vi "Tidy and package_v00.vi"(0 "OPO A":T2={"Offset Error"=-0.08983050847457627, "Gain Error"=1, "Offset DC"=-0.003954802259887008, "Gain DC"=1, "P Gain"=20, "P Bit Shift"=-12, "I Bit Shift"=-12, "I2 Bit Shift"=-27, "I Gain"=20, "I2 Gain"=0, "Lock Threshold"=45, "Lock"=FALSE, "Hold"=FALSE, "Scan Frequency"=10, "Scan Bit Shift"=-4, "DC negative"=FALSE, "Gains -ve "=FALSE} {"Scan Frequency" scale=1.0..30.0; "I2 Gain" scale=0.0..10.0; "I Gain" scale=0.0..50.0; "P Gain" scale=0.0..50.0; "Offset DC" scale=-0.1..0.1 scale format="%#_5f"; "Offset Error" scale=-0.1..0.1 scale format="%#_5f"}, 5 "OPO B":T2={"Offset Error"=0.0, "Gain Error"=1, "Offset DC"=1.0, "Gain DC"=1, "P Gain"=20, "P Bit Shift"=-12, "I Bit Shift"=-12, "I2 Bit Shift"=-27, "I Gain"=20, "I2 Gain"=0, "Lock Threshold"=29, "Lock"=FALSE, "Hold"=TRUE, "Scan Frequency"=11, "Scan Bit Shift"=-4, "DC negative"=FALSE, "Gains -ve "=TRUE} {"Scan Frequency" scale=1.0..30.0; "I2 Gain" scale=0.0..10.0; "I Gain" scale=0.0..50.0; "P Gain" scale=0.0..50.0; "Offset DC" scale=-0.1..0.1 scale format="%#_5f"; "Offset Error" scale=-0.1..0.1 scale format="%#_5f"}, 7 "MCC":T2={"Offset Error"=0.0, "Gain Error"=1, "Offset DC"=0.0, "Gain DC"=1, "P Gain"=10, "P Bit Shift"=-12, "I Bit Shift"=-12, "I2 Bit Shift"=-27, "I Gain"=10, "I2 Gain"=0, "Lock Threshold"=16, "Lock"=FALSE, "Hold"=TRUE, "Scan Frequency"=10, "Scan Bit Shift"=-4, "DC negative"=FALSE, "Gains -ve "=TRUE} {"Scan Frequency" scale=1.0..30.0; "I2 Gain" scale=0.0..10.0; "I Gain" scale=0.0..50.0; "P Gain" scale=0.0..50.0; "Offset DC" scale=-0.1..0.1 scale format="%#_5f"; "Offset Error" scale=-0.1..0.1 scale format="%#_5f"}, 9 "Doubler":T2={"Offset Error"=-0.014124293785310736, "Gain Error"=1, "Offset DC"=0.011864406779661016, "Gain DC"=1, "P Gain"=11, "P Bit Shift"=-12, "I Bit Shift"=-12, "I2 Bit Shift"=-27, "I Gain"=13, "I2 Gain"=0, "Lock Threshold"=24, "Lock"=FALSE, "Hold"=TRUE, "Scan Frequency"=12, "Scan Bit Shift"=-4, "DC negative"=FALSE, "Gains -ve "=TRUE} {"Scan Frequency" scale=1.0..30.0; "I2 Gain" scale=0.0..10.0; "I Gain" scale=0.0..50.0; "P Gain" scale=0.0..50.0; "Offset DC" scale=-0.1..0.1 scale format="%#_5f"; "Offset Error" scale=-0.1..0.1 scale format="%#_5f"}, 11 "PII Controls (-1)":T19={"Safety First"={"lim reset"=FALSE, "no limit"=FALSE, "pos slew rate * dt"=40, "neg slew rate * dt"=-5, "Hold All"=FALSE, "Count(Ticks)"=0}, "Error scale"={"Bit Shift"={"Bit Shift 1"=2, "Bit Shift 2"=0, "Bit Shift 3"=0, "Bit Shift 4"=0, "Bit Shift 5"=2, "Bit Shift 6"=0, "Bit Shift 7"=0, "Bit Shift 8"=0}, "Pre-Offset"={"Pre-Offset 1"=0, "Pre-Offset 2"=300, "Pre-Offset 3"=0, "Pre-Offset 4"=0, "Pre-Offset 5"=0, "Pre-Offset 6"=0, "Pre-Offset 7"=0, "Pre-Offset 8"=0}, "Post-Offset "={"Offset 1"=0, "Offset 2"=300, "Offset 3"=0, "Offset 4"=0, "Offset 5"=0, "Offset 6"=0, "Offset 7"=0, "Offset 8"=0}, "Gains"={"Gain 1"=5, "Gain 2"=5, "Gain 3"=0, "Gain 4"=0, "Gain 5"=0, "Gain 6"=0, "Gain 7"=0, "Gain 8"=0}, "Polarity DC"={"False 1"=FALSE, "False 2"=FALSE, "False 3"=FALSE, "False 4"=FALSE, "DC x -1"=FALSE, "DC x -1 2"=FALSE, "DC x -1 3"=FALSE, "DC x -1 4"=FALSE}}, "Lock Select"=enum."OPO A", "Controls"={"OPO A"={"Pre Offset"=0.0, "Offset"=0.0, "Gain"=0, "Bit Shift"=0, "Pre Offset 2"=0.0, "Offset 2"=0.0, "Gain 2"=0, "Bit Shift 2"=0, "P Gain"=0, "P Bit Shift"=0, "I Bit Shift"=0, "I2 Bit Shift"=0, "I Gain"=0, "I2 Gain"=0, "Lock Threshold"=0, "Lock"=FALSE, "Hold"=FALSE, "Scan Offset (mV)"=0.0, "Scan Amplitude (mV)"=0.0, "Scan Frequency"=0, "Scan Bit Shift"=0, "DC x -1"=FALSE, "Gains x -1"=FALSE, "I Max value"=0, "I2 Max value"=0}, "OPO B"={"Pre Offset"=0.0, "Offset"=0.0, "Gain"=0, "Bit Shift"=0, "Pre Offset 2"=0.0, "Offset 2"=0.0, "Gain 2"=0, "Bit Shift 2"=0, "P Gain"=0, "P Bit Shift"=0, "I Bit Shift"=0, "I2 Bit Shift"=0, "I Gain"=0, "I2 Gain"=0, "Lock Threshold"=0, "Lock"=FALSE, "Hold"=FALSE, "Scan Offset (mV)"=0.0, "Scan Amplitude (mV)"=0.0, "Scan Frequency"=0, "Scan Bit Shift"=0, "DC x -1"=FALSE, "Gains x -1"=FALSE, "I Max value"=0, "I2 Max value"=0}, "MCC"={"Pre Offset"=0.0, "Offset"=0.0, "Gain"=0, "Bit Shift"=0, "Pre Offset 2"=0.0, "Offset 2"=0.0, "Gain 2"=0, "Bit Shift 2"=0, "P Gain"=0, "P Bit Shift"=0, "I Bit Shift"=0, "I2 Bit Shift"=0, "I Gain"=0, "I2 Gain"=0, "Lock Threshold"=0, "Lock"=FALSE, "Hold"=FALSE, "Scan Offset (mV)"=0.0, "Scan Amplitude (mV)"=0.0, "Scan Frequency"=0, "Scan Bit Shift"=0, "DC x -1"=FALSE, "Gains x -1"=FALSE, "I Max value"=0, "I2 Max value"=0}, "Doubler"={"Pre Offset"=0.0, "Offset"=0.0, "Gain"=0, "Bit Shift"=0, "Pre Offset 2"=0.0, "Offset 2"=0.0, "Gain 2"=0, "Bit Shift 2"=0, "P Gain"=0, "P Bit Shift"=0, "I Bit Shift"=0, "I2 Bit Shift"=0, "I Gain"=0, "I2 Gain"=0, "Lock Threshold"=0, "Lock"=FALSE, "Hold"=FALSE, "Scan Offset (mV)"=0.0, "Scan Amplitude (mV)"=0.0, "Scan Frequency"=0, "Scan Bit Shift"=0, "DC x -1"=FALSE, "Gains x -1"=FALSE, "I Max value"=0, "I2 Max value"=0}}, "Scope IPs"={"Trigger Direction"=enum."either", "Trigger Delay (ms)"=0.0, "Aquisition Rate (kHz)"=1.0, "Trigger Offset (V)"=-1.0, "Trigger Channel"=0, "Channel Selector"={"Channel 1"=0, "Channel 2"=0, "Channel 3"=0, "Channel 4"=0}, "Scale Offset"={"Scaling"={"Scan Scale"=0, "Scan Scale 2"=0, "Scan Scale 3"=0, "Scan Scale 4"=0}, "Offset"={"Scan Offset"=0, "Scan Offset 2"=0, "Scan Offset 3"=0, "Scan Offset 4"=0}}}, "PII A"={"Lock"=FALSE, "Hold"=FALSE, "P Gain"=0, "P BS"=0, "I Gain"=0, "I BS"=0, "I2 G"=0, "I2 BS"=0, "Scan Amp"=0, "Scan Off"=0, "Scan FS"=0, "SFS BS"=0, "I Max value"=0, "I2 Max value"=0}, "PII B"={"Lock"=FALSE, "Hold"=FALSE, "P Gain"=0, "P BS"=0, "I Gain"=0, "I BS"=0, "I2 G"=0, "I2 BS"=0, "Scan Amp"=0, "Scan Off"=0, "Scan FS"=0, "SFS BS"=0, "I Max value"=0, "I2 Max value"=0}, "PII MCC"={"Lock"=FALSE, "Hold"=FALSE, "P Gain"=0, "P BS"=0, "I Gain"=0, "I BS"=0, "I2 G"=0, "I2 BS"=0, "Scan Amp"=0, "Scan Off"=0, "Scan FS"=0, "SFS BS"=0, "I Max value"=0, "I2 Max value"=0}, "PII Doubler"={"Lock"=FALSE, "Hold"=FALSE, "P Gain"=0, "P BS"=0, "I Gain"=0, "I BS"=0, "I2 G"=0, "I2 BS"=0, "Scan Amp"=0, "Scan Off"=0, "Scan FS"=0, "SFS BS"=0, "I Max value"=0, "I2 Max value"=0}, "Peak Depth (%)"={"Peak Depth (%) 1"=0, "Peak Depth (%) 2"=0, "Peak Depth (%) 3"=0, "Peak Depth (%) 4"=0}} {"Controls"."OPO A"."Scan Bit Shift" min=-8 max=0; "Controls"."OPO A"."Scan Frequency" scale=1.0..30.0; "Controls"."OPO A"."Scan Amplitude (mV)" scale=100.0..3000.0 scale format="%#_5f"; "Controls"."OPO A"."Scan Offset (mV)" scale=100.0..3000.0 scale format="%#_5f"; "Controls"."OPO A"."I2 Gain" scale=0.0..50.0; "Controls"."OPO A"."I Gain" scale=0.0..50.0; "Controls"."OPO A"."P Gain" scale=0.0..50.0; "Controls"."OPO A"."Offset 2" scale=-0.1..0.1 scale format="%#_5f"; "Controls"."OPO A"."Pre Offset 2" scale=-0.1..0.1 scale format="%#_5f"; "Controls"."OPO A"."Offset" scale=-0.1..0.1 scale format="%#_5f"; "Controls"."OPO A"."Pre Offset" scale=-0.1..0.1 scale format="%#_5f"; "Controls"."OPO B"."Scan Bit Shift" min=-8 max=0; "Controls"."OPO B"."Scan Frequency" scale=1.0..30.0; "Controls"."OPO B"."Scan Amplitude (mV)" scale=100.0..3000.0 scale format="%#_5f"; "Controls"."OPO B"."Scan Offset (mV)" scale=100.0..3000.0 scale format="%#_5f"; "Controls"."OPO B"."I2 Gain" scale=0.0..50.0; "Controls"."OPO B"."I Gain" scale=0.0..50.0; "Controls"."OPO B"."P Gain" scale=0.0..50.0; "Controls"."OPO B"."Offset 2" scale=-0.1..0.1 scale format="%#_5f"; "Controls"."OPO B"."Pre Offset 2" scale=-0.1..0.1 scale format="%#_5f"; "Controls"."OPO B"."Offset" scale=-0.1..0.1 scale format="%#_5f"; "Controls"."OPO B"."Pre Offset" scale=-0.1..0.1 scale format="%#_5f"; "Controls"."MCC"."Scan Bit Shift" min=-8 max=0; "Controls"."MCC"."Scan Frequency" scale=1.0..30.0; "Controls"."MCC"."Scan Amplitude (mV)" scale=100.0..3000.0 scale format="%#_5f"; "Controls"."MCC"."Scan Offset (mV)" scale=100.0..3000.0 scale format="%#_5f"; "Controls"."MCC"."I2 Gain" scale=0.0..50.0; "Controls"."MCC"."I Gain" scale=0.0..50.0; "Controls"."MCC"."P Gain" scale=0.0..50.0; "Controls"."MCC"."Offset 2" scale=-0.1..0.1 scale format="%#_5f"; "Controls"."MCC"."Pre Offset 2" scale=-0.1..0.1 scale format="%#_5f"; "Controls"."MCC"."Offset" scale=-0.1..0.1 scale format="%#_5f"; "Controls"."MCC"."Pre Offset" scale=-0.1..0.1 scale format="%#_5f"; "Controls"."Doubler"."Scan Bit Shift" min=-8 max=0; "Controls"."Doubler"."Scan Frequency" scale=1.0..30.0; "Controls"."Doubler"."Scan Amplitude (mV)" scale=100.0..3000.0 scale format="%#_5f"; "Controls"."Doubler"."Scan Offset (mV)" scale=100.0..3000.0 scale format="%#_5f"; "Controls"."Doubler"."I2 Gain" scale=0.0..50.0; "Controls"."Doubler"."I Gain" scale=0.0..50.0; "Controls"."Doubler"."P Gain" scale=0.0..50.0; "Controls"."Doubler"."Offset 2" scale=-0.1..0.1 scale format="%#_5f"; "Controls"."Doubler"."Pre Offset 2" scale=-0.1..0.1 scale format="%#_5f"; "Controls"."Doubler"."Offset" scale=-0.1..0.1 scale format="%#_5f"; "Controls"."Doubler"."Pre Offset" scale=-0.1..0.1 scale format="%#_5f"}, 12 "Cavity Extras":T16={"Pre-Offset"={"OPO A"=0.0, "OPO B"=0.0, "MCC"=0.0, "Doubler"=0.0}, "Pre-Offset DC"={"OPO A"=0.0, "OPO B"=0.0, "MCC"=0.0, "Doubler"=0.0}, "I Max value"=20000, "I2 Max value"=20000, "Scan Offset"={"OPO A"=0.0, "OPO B"=0.0, "MCC"=0.0, "Doubler"=0.0}, "Scan Ampl."={"OPO A"=1000.0, "OPO B"=1000.0, "MCC"=1000.0, "Doubler"=1000.0}, "Scan-PII thresh"={"OPO A"=0, "OPO B"=0, "MCC"=0, "Doubler"=0}, "Re-Scan thresh"={"OPO A"=0, "OPO B"=0, "MCC"=0, "Doubler"=0}}, 13 "Scope+Safety":T15={"Safety First"={"lim reset"=FALSE, "no limit"=FALSE, "pos slew rate * dt"=100, "neg slew rate * dt"=-100, "Count(Ticks)"=0}, "Scope IPs"={"Trigger Direction"=enum."minus-plus", "Trigger Delay (ms)"=0.0, "Aquisition Rate (kHz)"=4000.0, "Trigger Offset (V)"=0.0, "Scale Offset"={"Scaling"={"Error signal"=1, "Output"=1, "DC Monitor"=1, "Threshold"=1}, "Offset"={"Error Signal"=0, "Output"=0, "DC Monitor"=0, "Threshold"=0}}}}, 14 "Hold All":T12) -> (3 "PII Controls cluster":T19={"Safety First"={"lim reset"=FALSE, "no limit"=FALSE, "pos slew rate * dt"=40, "neg slew rate * dt"=-5, "Hold All"=FALSE, "Count(Ticks)"=0}, "Error scale"={"Bit Shift"={"Bit Shift 1"=2, "Bit Shift 2"=0, "Bit Shift 3"=0, "Bit Shift 4"=0, "Bit Shift 5"=2, "Bit Shift 6"=0, "Bit Shift 7"=0, "Bit Shift 8"=0}, "Pre-Offset"={"Pre-Offset 1"=0, "Pre-Offset 2"=300, "Pre-Offset 3"=0, "Pre-Offset 4"=0, "Pre-Offset 5"=0, "Pre-Offset 6"=0, "Pre-Offset 7"=0, "Pre-Offset 8"=0}, "Post-Offset "={"Offset 1"=0, "Offset 2"=300, "Offset 3"=0, "Offset 4"=0, "Offset 5"=0, "Offset 6"=0, "Offset 7"=0, "Offset 8"=0}, "Gains"={"Gain 1"=5, "Gain 2"=5, "Gain 3"=0, "Gain 4"=0, "Gain 5"=0, "Gain 6"=0, "Gain 7"=0, "Gain 8"=0}, "Polarity DC"={"False 1"=FALSE, "False 2"=FALSE, "False 3"=FALSE, "False 4"=FALSE, "DC x -1"=FALSE, "DC x -1 2"=FALSE, "DC x -1 3"=FALSE, "DC x -1 4"=FALSE}}, "Lock Select"=enum."OPO A", "Controls"={"OPO A"={"Pre Offset"=0.0, "Offset"=0.0, "Gain"=0, "Bit Shift"=0, "Pre Offset 2"=0.0, "Offset 2"=0.0, "Gain 2"=0, "Bit Shift 2"=0, "P Gain"=0, "P Bit Shift"=0, "I Bit Shift"=0, "I2 Bit Shift"=0, "I Gain"=0, "I2 Gain"=0, "Lock Threshold"=0, "Lock"=FALSE, "Hold"=FALSE, "Scan Offset (mV)"=0.0, "Scan Amplitude (mV)"=0.0, "Scan Frequency"=0, "Scan Bit Shift"=0, "DC x -1"=FALSE, "Gains x -1"=FALSE, "I Max value"=0, "I2 Max value"=0}, "OPO B"={"Pre Offset"=0.0, "Offset"=0.0, "Gain"=0, "Bit Shift"=0, "Pre Offset 2"=0.0, "Offset 2"=0.0, "Gain 2"=0, "Bit Shift 2"=0, "P Gain"=0, "P Bit Shift"=0, "I Bit Shift"=0, "I2 Bit Shift"=0, "I Gain"=0, "I2 Gain"=0, "Lock Threshold"=0, "Lock"=FALSE, "Hold"=FALSE, "Scan Offset (mV)"=0.0, "Scan Amplitude (mV)"=0.0, "Scan Frequency"=0, "Scan Bit Shift"=0, "DC x -1"=FALSE, "Gains x -1"=FALSE, "I Max value"=0, "I2 Max value"=0}, "MCC"={"Pre Offset"=0.0, "Offset"=0.0, "Gain"=0, "Bit Shift"=0, "Pre Offset 2"=0.0, "Offset 2"=0.0, "Gain 2"=0, "Bit Shift 2"=0, "P Gain"=0, "P Bit Shift"=0, "I Bit Shift"=0, "I2 Bit Shift"=0, "I Gain"=0, "I2 Gain"=0, "Lock Threshold"=0, "Lock"=FALSE, "Hold"=FALSE, "Scan Offset (mV)"=0.0, "Scan Amplitude (mV)"=0.0, "Scan Frequency"=0, "Scan Bit Shift"=0, "DC x -1"=FALSE, "Gains x -1"=FALSE, "I Max value"=0, "I2 Max value"=0}, "Doubler"={"Pre Offset"=0.0, "Offset"=0.0, "Gain"=0, "Bit Shift"=0, "Pre Offset 2"=0.0, "Offset 2"=0.0, "Gain 2"=0, "Bit Shift 2"=0, "P Gain"=0, "P Bit Shift"=0, "I Bit Shift"=0, "I2 Bit Shift"=0, "I Gain"=0, "I2 Gain"=0, "Lock Threshold"=0, "Lock"=FALSE, "Hold"=FALSE, "Scan Offset (mV)"=0.0, "Scan Amplitude (mV)"=0.0, "Scan Frequency"=0, "Scan Bit Shift"=0, "DC x -1"=FALSE, "Gains x -1"=FALSE, "I Max value"=0, "I2 Max value"=0}}, "Scope IPs"={"Trigger Direction"=enum."either", "Trigger Delay (ms)"=0.0, "Aquisition Rate (kHz)"=1.0, "Trigger Offset (V)"=-1.0, "Trigger Channel"=0, "Channel Selector"={"Channel 1"=0, "Channel 2"=0, "Channel 3"=0, "Channel 4"=0}, "Scale Offset"={"Scaling"={"Scan Scale"=0, "Scan Scale 2"=0, "Scan Scale 3"=0, "Scan Scale 4"=0}, "Offset"={"Scan Offset"=0, "Scan Offset 2"=0, "Scan Offset 3"=0, "Scan Offset 4"=0}}}, "PII A"={"Lock"=FALSE, "Hold"=FALSE, "P Gain"=0, "P BS"=0, "I Gain"=0, "I BS"=0, "I2 G"=0, "I2 BS"=0, "Scan Amp"=0, "Scan Off"=0, "Scan FS"=0, "SFS BS"=0, "I Max value"=0, "I2 Max value"=0}, "PII B"={"Lock"=FALSE, "Hold"=FALSE, "P Gain"=0, "P BS"=0, "I Gain"=0, "I BS"=0, "I2 G"=0, "I2 BS"=0, "Scan Amp"=0, "Scan Off"=0, "Scan FS"=0, "SFS BS"=0, "I Max value"=0, "I2 Max value"=0}, "PII MCC"={"Lock"=FALSE, "Hold"=FALSE, "P Gain"=0, "P BS"=0, "I Gain"=0, "I BS"=0, "I2 G"=0, "I2 BS"=0, "Scan Amp"=0, "Scan Off"=0, "Scan FS"=0, "SFS BS"=0, "I Max value"=0, "I2 Max value"=0}, "PII Doubler"={"Lock"=FALSE, "Hold"=FALSE, "P Gain"=0, "P BS"=0, "I Gain"=0, "I BS"=0, "I2 G"=0, "I2 BS"=0, "Scan Amp"=0, "Scan Off"=0, "Scan FS"=0, "SFS BS"=0, "I Max value"=0, "I2 Max value"=0}, "Peak Depth (%)"={"Peak Depth (%) 1"=0, "Peak Depth (%) 2"=0, "Peak Depth (%) 3"=0, "Peak Depth (%) 4"=0}} {"Controls"."OPO A"."Scan Bit Shift" min=-8 max=0; "Controls"."OPO A"."Scan Frequency" scale=1.0..30.0; "Controls"."OPO A"."Scan Amplitude (mV)" scale=100.0..3000.0 scale format="%#_5f"; "Controls"."OPO A"."Scan Offset (mV)" scale=100.0..3000.0 scale format="%#_5f"; "Controls"."OPO A"."I2 Gain" scale=0.0..50.0; "Controls"."OPO A"."I Gain" scale=0.0..50.0; "Controls"."OPO A"."P Gain" scale=0.0..50.0; "Controls"."OPO A"."Offset 2" scale=-0.1..0.1 scale format="%#_5f"; "Controls"."OPO A"."Pre Offset 2" scale=-0.1..0.1 scale format="%#_5f"; "Controls"."OPO A"."Offset" scale=-0.1..0.1 scale format="%#_5f"; "Controls"."OPO A"."Pre Offset" scale=-0.1..0.1 scale format="%#_5f"; "Controls"."OPO B"."Scan Bit Shift" min=-8 max=0; "Controls"."OPO B"."Scan Frequency" scale=1.0..30.0; "Controls"."OPO B"."Scan Amplitude (mV)" scale=100.0..3000.0 scale format="%#_5f"; "Controls"."OPO B"."Scan Offset (mV)" scale=100.0..3000.0 scale format="%#_5f"; "Controls"."OPO B"."I2 Gain" scale=0.0..50.0; "Controls"."OPO B"."I Gain" scale=0.0..50.0; "Controls"."OPO B"."P Gain" scale=0.0..50.0; "Controls"."OPO B"."Offset 2" scale=-0.1..0.1 scale format="%#_5f"; "Controls"."OPO B"."Pre Offset 2" scale=-0.1..0.1 scale format="%#_5f"; "Controls"."OPO B"."Offset" scale=-0.1..0.1 scale format="%#_5f"; "Controls"."OPO B"."Pre Offset" scale=-0.1..0.1 scale format="%#_5f"; "Controls"."MCC"."Scan Bit Shift" min=-8 max=0; "Controls"."MCC"."Scan Frequency" scale=1.0..30.0; "Controls"."MCC"."Scan Amplitude (mV)" scale=100.0..3000.0 scale format="%#_5f"; "Controls"."MCC"."Scan Offset (mV)" scale=100.0..3000.0 scale format="%#_5f"; "Controls"."MCC"."I2 Gain" scale=0.0..50.0; "Controls"."MCC"."I Gain" scale=0.0..50.0; "Controls"."MCC"."P Gain" scale=0.0..50.0; "Controls"."MCC"."Offset 2" scale=-0.1..0.1 scale format="%#_5f"; "Controls"."MCC"."Pre Offset 2" scale=-0.1..0.1 scale format="%#_5f"; "Controls"."MCC"."Offset" scale=-0.1..0.1 scale format="%#_5f"; "Controls"."MCC"."Pre Offset" scale=-0.1..0.1 scale format="%#_5f"; "Controls"."Doubler"."Scan Bit Shift" min=-8 max=0; "Controls"."Doubler"."Scan Frequency" scale=1.0..30.0; "Controls"."Doubler"."Scan Amplitude (mV)" scale=100.0..3000.0 scale format="%#_5f"; "Controls"."Doubler"."Scan Offset (mV)" scale=100.0..3000.0 scale format="%#_5f"; "Controls"."Doubler"."I2 Gain" scale=0.0..50.0; "Controls"."Doubler"."I Gain" scale=0.0..50.0; "Controls"."Doubler"."P Gain" scale=0.0..50.0; "Controls"."Doubler"."Offset 2" scale=-0.1..0.1 scale format="%#_5f"; "Controls"."Doubler"."Pre Offset 2" scale=-0.1..0.1 scale format="%#_5f"; "Controls"."Doubler"."Offset" scale=-0.1..0.1 scale format="%#_5f"; "Controls"."Doubler"."Pre Offset" scale=-0.1..0.1 scale format="%#_5f"}, 4 "Scope IPs":T13, 15 "Control to FPGA":T18)   [LabVIEW 2010]
doc: "The data structures from the User Interface need are rebundled here to match that of the FPGA_Cavity VI."
uses:
  Strict Type Defs/Top Level Control.ctl
  Strict Type Defs/Safety First.ctl
  Strict Type Defs/Error_Scale.ctl
  Strict Type Defs/Control GUI v00.ctl
  Strict Type Defs/Slider and display.ctl
  Strict Type Defs/I16 white control.ctl
  Strict Type Defs/PII Gains.ctl
  Strict Type Defs/Thresh slider.ctl
  Strict Type Defs/Lock or Hold.ctl
  Strict Type Defs/Scan Amp slider.ctl
  Strict Type Defs/Scan Frequency.ctl
  Strict Type Defs/DC polarity.ctl
  Strict Type Defs/Gains negative.ctl
  Strict Type Defs/I max value.ctl
  Strict Type Defs/Top Level PII.ctl
  Strict Type Defs/Control GUI v01.ctl
  Strict Type Defs/I2 gain slider.ctl
  Strict Type Defs/Scan Freq Slider.ctl
  Strict Type Defs/Gains negative vertical.ctl
  Strict Type Defs/Cavity Extras.ctl
  Strict Type Defs/Pre-Offset.ctl
  Strict Type Defs/Scope and Safety.ctl
  Strict Type Defs/Hold All.ctl
  Strict Type Defs/Lock Select 4.ctl
panel:
  in  "Lock 4":T1
  in  "Safety First":T14
  in  "Control":T18
  # "PII Gains"
  # "Lock"
  # "Error Signal"
  # "Monitor"
  # "Scan"
  # "DC positive"
  # "PII Gains"
  # "Lock"
  # "Error Signal"
  # "Monitor"
  # "Scan"
  # "DC positive"
  # "PII Gains"
  # "Lock"
  # "Error Signal"
  # "Monitor"
  # "Scan"
  # "DC positive"
  # "PII Gains"
  # "Lock"
  # "Error Signal"
  # "Monitor"
  # "Scan"
  # "DC positive"
  # "Error Signal"
  # "Cavity Monitors"
  # "PII Gains"
  # "Lock"
  # "Scan"
  # "Error Signal"
  # "Cavity Monitors"
  # "PII Gains"
  # "Lock"
  # "Scan"
  # "Error Signal"
  # "Cavity Monitors"
  # "PII Gains"
  # "Lock"
  # "Scan"
  # "Error Signal"
  # "Cavity Monitors"
  # "PII Gains"
  # "Lock"
  # "Scan"
  # "Error Signal"
  # "Cavity Monitors"
  # "PII Gains"
  # "Lock"
  # "Scan"
  # "Error Signal"
  # "Cavity Monitors"
  # "PII Gains"
  # "Lock"
  # "Scan"
  # "Error Signal"
  # "Cavity Monitors"
  # "PII Gains"
  # "Lock"
  # "Scan"
  # "Error Signal"
  # "Cavity Monitors"
  # "PII Gains"
  # "Lock"
  # "Scan"
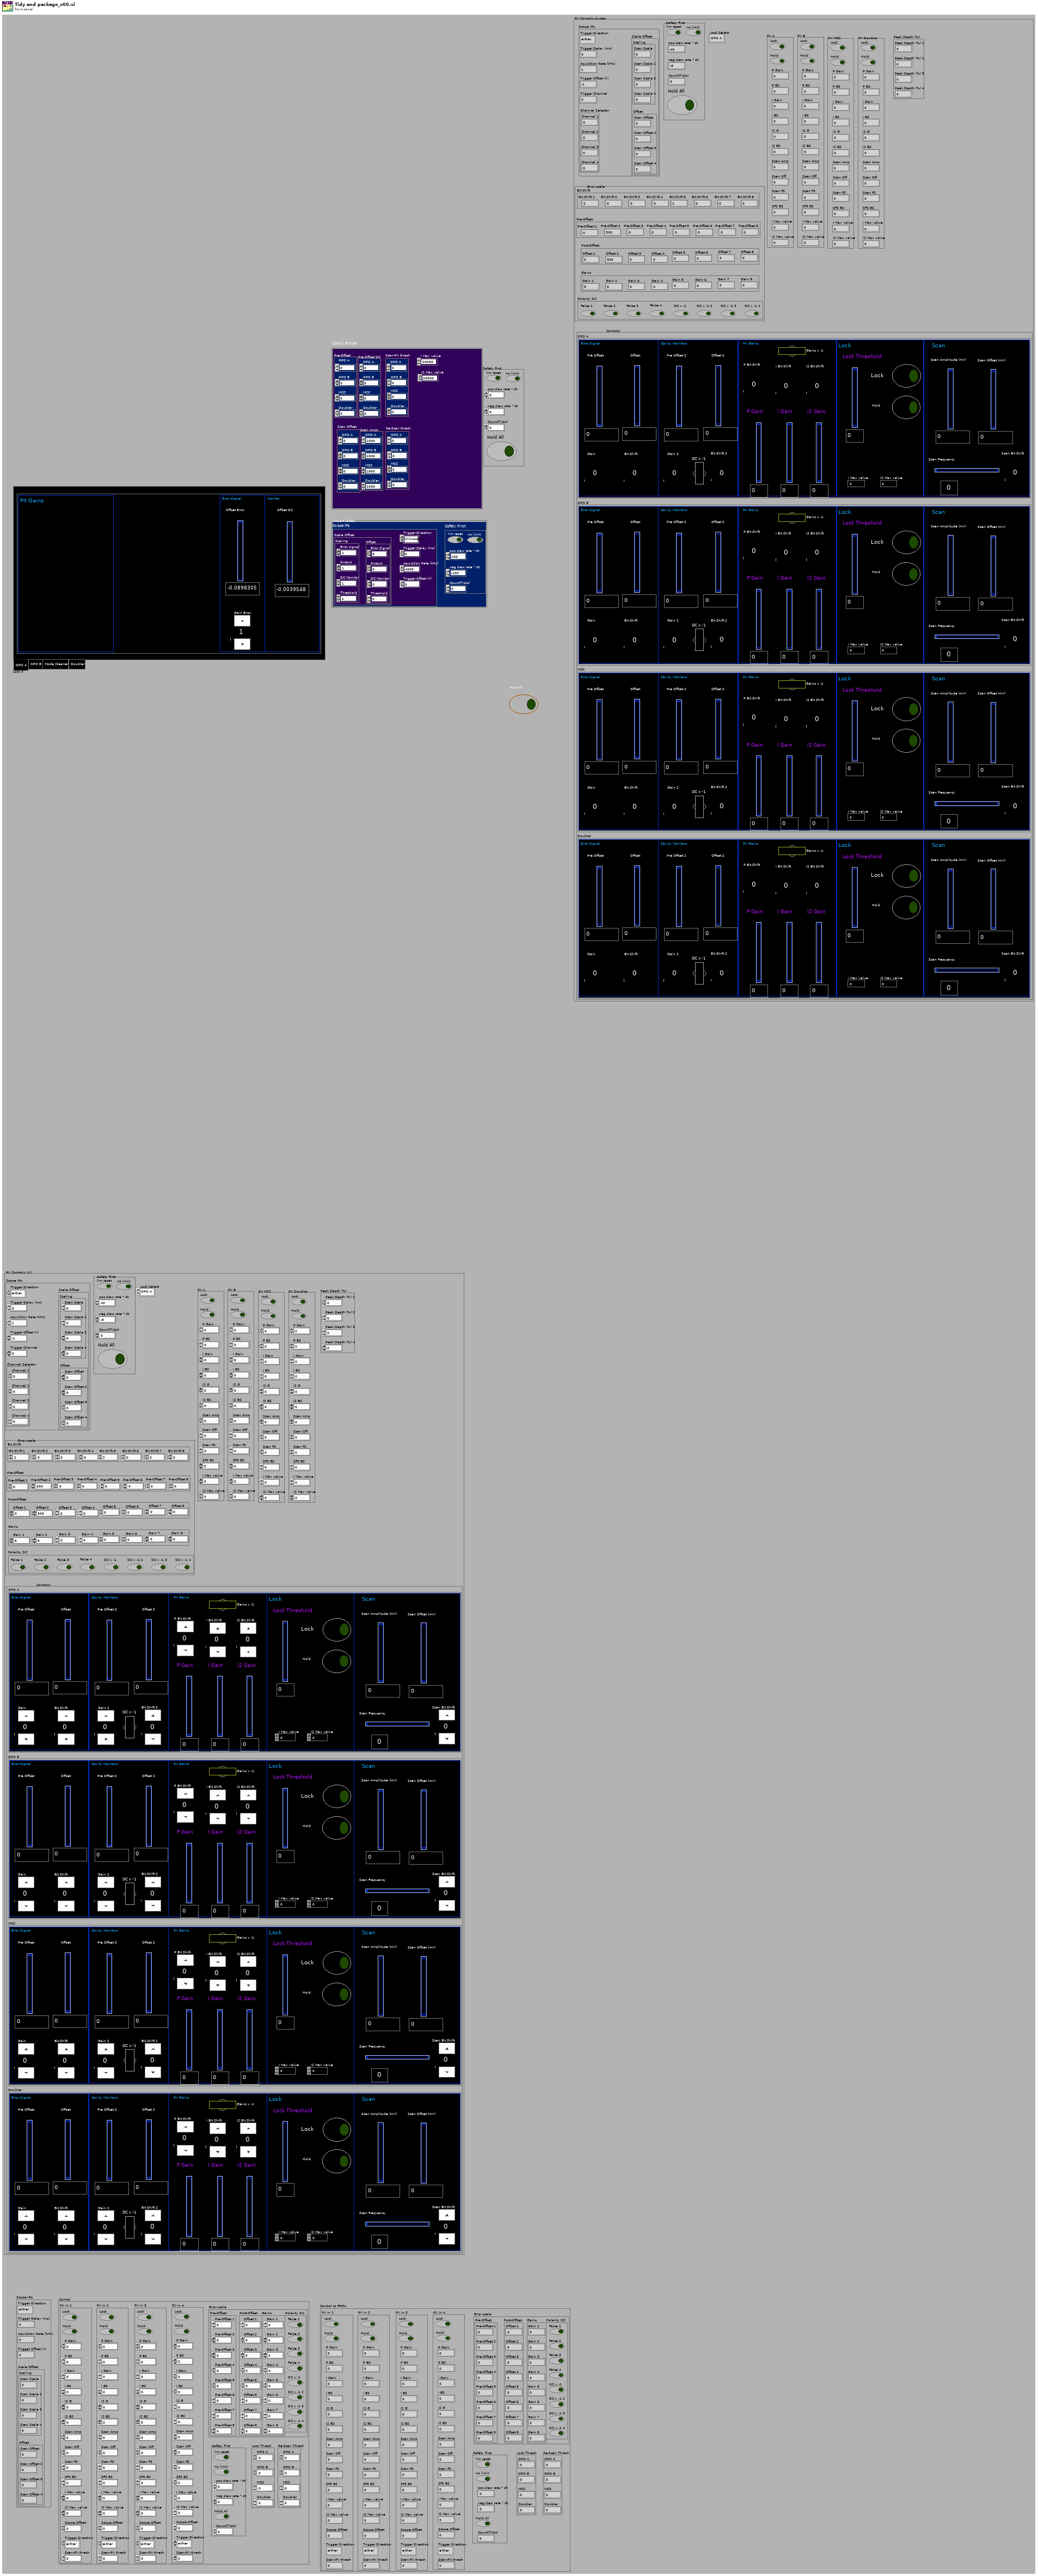
[diagram p1: front panel]
types:
  T1 = typedef "Lock Select 4.ctl" = enum32{"OPO A", "OPO B", "Mode Cleaner", "Doubler"}
  T2 = typedef "Control GUI v01.ctl" = cluster{"Offset Error":T3, "Gain Error":T4, "Offset DC":T3, "Gain DC":T4, "P Gain":T5, "P Bit Shift":T4, "I Bit Shift":T4, "I2 Bit Shift":T4, "I Gain":T5, "I2 Gain":T6, "Lock Threshold":T7, "Lock":T8, "Hold":T8, "Scan Frequency":T9, "Scan Bit Shift":T4, "DC negative":T10, "Gains -ve ":T11}
  T3 = typedef "Slider and display.ctl" = dbl
  T4 = typedef "I16 white control.ctl" = i16
  T5 = typedef "PII Gains.ctl" = i32
  T6 = typedef "I2 gain slider.ctl" = i32
  T7 = typedef "Thresh slider.ctl" = i16
  T8 = typedef "Lock or Hold.ctl" = bool
  T9 = typedef "Scan Freq Slider.ctl" = u16
  T10 = typedef "DC polarity.ctl" = bool
  T11 = typedef "Gains negative vertical.ctl" = bool
  T12 = typedef "Hold All.ctl" = bool
  T13 = cluster{"Trigger Direction":enum8{"either", "minus-plus", "plus-minus"}, "Trigger Delay (ms)":dbl, "Aquisition Rate (kHz)":dbl, "Trigger Offset (V)":dbl, "Scale Offset":cluster{"Scaling":cluster{"Scan Scale":i16, "Scan Scale 2":i16, "Scan Scale 3":i16, "Scan Scale 4":i16}, "Offset":cluster{"Scan Offset":i16, "Scan Offset 2":i16, "Scan Offset 3":i16, "Scan Offset 4":i16}}}
  T14 = typedef "Safety First.ctl" = cluster{"lim reset":bool, "no limit":bool, "pos slew rate * dt":i16, "neg slew rate * dt":i16, "Hold All":bool, "Count(Ticks)":u32}
  T15 = typedef "Scope and Safety.ctl" = cluster{"Safety First":cluster{"lim reset":bool, "no limit":bool, "pos slew rate * dt":i16, "neg slew rate * dt":i16, "Count(Ticks)":u32}, "Scope IPs":cluster{"Trigger Direction":enum8{"either", "minus-plus", "plus-minus"}, "Trigger Delay (ms)":dbl, "Aquisition Rate (kHz)":dbl, "Trigger Offset (V)":dbl, "Scale Offset":cluster{"Scaling":cluster{"Error signal":i16, "Output":i16, "DC Monitor":i16, "Threshold":i16}, "Offset":cluster{"Error Signal":i16, "Output":i16, "DC Monitor":i16, "Threshold":i16}}}}
  T16 = typedef "Cavity Extras.ctl" = cluster{"Pre-Offset":T17, "Pre-Offset DC":T17, "I Max value":i32, "I2 Max value":i32, "Scan Offset":T17, "Scan Ampl.":T17, "Scan-PII thresh":cluster{"OPO A":i16, "OPO B":i16, "MCC":i16, "Doubler":i16}, "Re-Scan thresh":cluster{"OPO A":i16, "OPO B":i16, "MCC":i16, "Doubler":i16}}
  T17 = typedef "Pre-Offset.ctl" = cluster{"OPO A":dbl, "OPO B":dbl, "MCC":dbl, "Doubler":dbl}
  T18 = cluster{"PII In 1":cluster{"Lock":bool, "Hold":bool, "P Gain":i32, "P BS":i16, "I Gain":i32, "I BS":i16, "I2 G":i32, "I2 BS":i16, "Scan Amp":i16, "Scan Off":i16, "Scan FS":u16, "SFS BS":i16, "I Max value":i32, "I2 Max value":i32, "Scope.Offset":i16, "Trigger Direction":enum8{"either", "minus-plus", "plus-minus"}, "Scan-PII thresh":i16}, "PII In 2":cluster{"Lock":bool, "Hold":bool, "P Gain":i32, "P BS":i16, "I Gain":i32, "I BS":i16, "I2 G":i32, "I2 BS":i16, "Scan Amp":i16, "Scan Off":i16, "Scan FS":u16, "SFS BS":i16, "I Max value":i32, "I2 Max value":i32, "Scope.Offset":i16, "Trigger Direction":enum8{"either", "minus-plus", "plus-minus"}, "Scan-PII thresh":i16}, "PII In 3":cluster{"Lock":bool, "Hold":bool, "P Gain":i32, "P BS":i16, "I Gain":i32, "I BS":i16, "I2 G":i32, "I2 BS":i16, "Scan Amp":i16, "Scan Off":i16, "Scan FS":u16, "SFS BS":i16, "I Max value":i32, "I2 Max value":i32, "Scope.Offset":i16, "Trigger Direction":enum8{"either", "minus-plus", "plus-minus"}, "Scan-PII thresh":i16}, "PII In 4":cluster{"Lock":bool, "Hold":bool, "P Gain":i32, "P BS":i16, "I Gain":i32, "I BS":i16, "I2 G":i32, "I2 BS":i16, "Scan Amp":i16, "Scan Off":i16, "Scan FS":u16, "SFS BS":i16, "I Max value":i32, "I2 Max value":i32, "Scope.Offset":i16, "Trigger Direction":enum8{"either", "minus-plus", "plus-minus"}, "Scan-PII thresh":i16}, "Safety First":cluster{"lim reset":bool, "no limit":bool, "pos slew rate * dt":i16, "neg slew rate * dt":i16, "Hold All":bool, "Count(Ticks)":u32}, "Error scale":cluster{"Pre-Offset":cluster{"Pre-Offset 1":i16, "Pre-Offset 2":i16, "Pre-Offset 3":i16, "Pre-Offset 4":i16, "Pre-Offset 5":i16, "Pre-Offset 6":i16, "Pre-Offset 7":i16, "Pre-Offset 8":i16}, "Post-Offset ":cluster{"Offset 1":i16, "Offset 2":i16, "Offset 3":i16, "Offset 4":i16, "Offset 5":i16, "Offset 6":i16, "Offset 7":i16, "Offset 8":i16}, "Gains":cluster{"Gain 1":i16, "Gain 2":i16, "Gain 3":i16, "Gain 4":i16, "Gain 5":i16, "Gain 6":i16, "Gain 7":i16, "Gain 8":i16}, "Polarity DC":cluster{"False 1":bool, "False 2":bool, "False 3":bool, "False 4":bool, "DC x -1":bool, "DC x -1 2":bool, "DC x -1 3":bool, "DC x -1 4":bool}}, "Lock Thresh":cluster{"OPO A":i16, "OPO B":i16, "MCC":i16, "Doubler":i16}, "Re-Scan Thresh":cluster{"OPO A":i16, "OPO B":i16, "MCC":i16, "Doubler":i16}}
  T19 = typedef "Top Level Control.ctl" = cluster{"Safety First":T14, "Error scale":T20, "Lock Select":enum32{"OPO A", "OPO B", "Mode Cleaner", "Doubler", "パラメ OPO A", "パラメ OPO B", "EPR Beamsplitter", "Graph Beamsplitter", "Homodyne A", "Homodyne B"}, "Controls":cluster{"OPO A":T21, "OPO B":T21, "MCC":T21, "Doubler":T21}, "Scope IPs":cluster{"Trigger Direction":enum8{"either", "minus-plus", "plus-minus"}, "Trigger Delay (ms)":dbl, "Aquisition Rate (kHz)":dbl, "Trigger Offset (V)":dbl, "Trigger Channel":i32, "Channel Selector":cluster{"Channel 1":i32, "Channel 2":i32, "Channel 3":i32, "Channel 4":i32}, "Scale Offset":cluster{"Scaling":cluster{"Scan Scale":i16, "Scan Scale 2":i16, "Scan Scale 3":i16, "Scan Scale 4":i16}, "Offset":cluster{"Scan Offset":i16, "Scan Offset 2":i16, "Scan Offset 3":i16, "Scan Offset 4":i16}}}, "PII A":T26, "PII B":T26, "PII MCC":T26, "PII Doubler":T26, "Peak Depth (%)":cluster{"Peak Depth (%) 1":i16, "Peak Depth (%) 2":i16, "Peak Depth (%) 3":i16, "Peak Depth (%) 4":i16}}
  T20 = typedef "Error_Scale.ctl" = cluster{"Bit Shift":cluster{"Bit Shift 1":i16, "Bit Shift 2":i16, "Bit Shift 3":i16, "Bit Shift 4":i16, "Bit Shift 5":i16, "Bit Shift 6":i16, "Bit Shift 7":i16, "Bit Shift 8":i16}, "Pre-Offset":cluster{"Pre-Offset 1":i16, "Pre-Offset 2":i16, "Pre-Offset 3":i16, "Pre-Offset 4":i16, "Pre-Offset 5":i16, "Pre-Offset 6":i16, "Pre-Offset 7":i16, "Pre-Offset 8":i16}, "Post-Offset ":cluster{"Offset 1":i16, "Offset 2":i16, "Offset 3":i16, "Offset 4":i16, "Offset 5":i16, "Offset 6":i16, "Offset 7":i16, "Offset 8":i16}, "Gains":cluster{"Gain 1":i16, "Gain 2":i16, "Gain 3":i16, "Gain 4":i16, "Gain 5":i16, "Gain 6":i16, "Gain 7":i16, "Gain 8":i16}, "Polarity DC":cluster{"False 1":bool, "False 2":bool, "False 3":bool, "False 4":bool, "DC x -1":bool, "DC x -1 2":bool, "DC x -1 3":bool, "DC x -1 4":bool}}
  T21 = typedef "Control GUI v00.ctl" = cluster{"Pre Offset":T3, "Offset":T3, "Gain":T4, "Bit Shift":T4, "Pre Offset 2":T3, "Offset 2":T3, "Gain 2":T4, "Bit Shift 2":T4, "P Gain":T5, "P Bit Shift":T4, "I Bit Shift":T4, "I2 Bit Shift":T4, "I Gain":T5, "I2 Gain":T5, "Lock Threshold":T7, "Lock":T8, "Hold":T8, "Scan Offset (mV)":T22, "Scan Amplitude (mV)":T22, "Scan Frequency":T23, "Scan Bit Shift":T4, "DC x -1":T10, "Gains x -1":T24, "I Max value":T25, "I2 Max value":T25}
  T22 = typedef "Scan Amp slider.ctl" = dbl
  T23 = typedef "Scan Frequency.ctl" = u16
  T24 = typedef "Gains negative.ctl" = bool
  T25 = typedef "I max value.ctl" = i16
  T26 = typedef "Top Level PII.ctl" = cluster{"Lock":bool, "Hold":bool, "P Gain":i16, "P BS":i16, "I Gain":i16, "I BS":i16, "I2 G":i16, "I2 BS":i16, "Scan Amp":i16, "Scan Off":i16, "Scan FS":u16, "SFS BS":i16, "I Max value":i16, "I2 Max value":i16}
  T27 = enum32{"OPO A", "OPO B", "Mode Cleaner", "Doubler", "パラメ OPO A", "パラメ OPO B", "EPR Beamsplitter", "Graph Beamsplitter", "Homodyne A", "Homodyne B"}
  T28 = typedef "Extras PII.ctl" = cluster{"Pre-Offset":dbl, "Pre-Offset DC":dbl, "Scan Offset":dbl, "Scan Amplitude":dbl, "Scan-PII thresh":i16, "Re-Scan Thresh":i16, "I Max value":i32, "I2 Max value":i32, "Trigger Direction":enum8{"either", "minus-plus", "plus-minus"}, "Trigger Offset (V)":dbl}
  T29 = typedef "Controls Converted.ctl" = cluster{"Error individual":T30, "PII cavity":T31, "Lock Thresh":i16, "Re-Scan Thresh":i16}
  T30 = typedef "Errors Converted.ctl" = cluster{"Error Pre Offset":i16, "Error Offset":i16, "DC Pre Offset":i16, "DC Offset":i16, "Polarity DC":bool, "Error Gain":i16, "DC Gain":i16}
  T31 = typedef "PII individual.ctl" = cluster{"Lock":bool, "Hold":bool, "P Gain":i32, "P BS":i16, "I Gain":i32, "I BS":i16, "I2 G":i32, "I2 BS":i16, "Scan Amp":i16, "Scan Off":i16, "Scan FS":u16, "SFS BS":i16, "I Max value":i32, "I2 Max value":i32, "Scope.Offset":i16, "Trigger Direction":enum8{"either", "minus-plus", "plus-minus"}, "Scan-PII thresh":i16}
  T32 = cluster{"Trigger Direction":enum8{"either", "minus-plus", "plus-minus"}, "Trigger Delay (ms)":dbl, "Aquisition Rate (kHz)":dbl, "Trigger Offset (V)":dbl, "Scale Offset":cluster{"Scaling":cluster{"Error signal":i16, "Output":i16, "DC Monitor":i16, "Threshold":i16}, "Offset":cluster{"Error Signal":i16, "Output":i16, "DC Monitor":i16, "Threshold":i16}}}
  T33 = cluster{"Lock":cluster{"OPO A":i16, "OPO B":i16, "MCC":i16, "Doubler":i16}, "Re-Scan":cluster{"OPO A":i16, "OPO B":i16, "MCC":i16, "Doubler":i16}}
  T34 = typedef "Error Scale.ctl" = cluster{"Pre-Offset":cluster{"Pre-Offset 1":i16, "Pre-Offset 2":i16, "Pre-Offset 3":i16, "Pre-Offset 4":i16, "Pre-Offset 5":i16, "Pre-Offset 6":i16, "Pre-Offset 7":i16, "Pre-Offset 8":i16}, "Post-Offset ":cluster{"Offset 1":i16, "Offset 2":i16, "Offset 3":i16, "Offset 4":i16, "Offset 5":i16, "Offset 6":i16, "Offset 7":i16, "Offset 8":i16}, "Gains":cluster{"Gain 1":i16, "Gain 2":i16, "Gain 3":i16, "Gain 4":i16, "Gain 5":i16, "Gain 6":i16, "Gain 7":i16, "Gain 8":i16}, "Polarity DC":cluster{"False 1":bool, "False 2":bool, "False 3":bool, "False 4":bool, "DC x -1":bool, "DC x -1 2":bool, "DC x -1 3":bool, "DC x -1 4":bool}}
  T35 = cluster{"OPO A":i16, "OPO B":i16, "MCC":i16, "Doubler":i16}
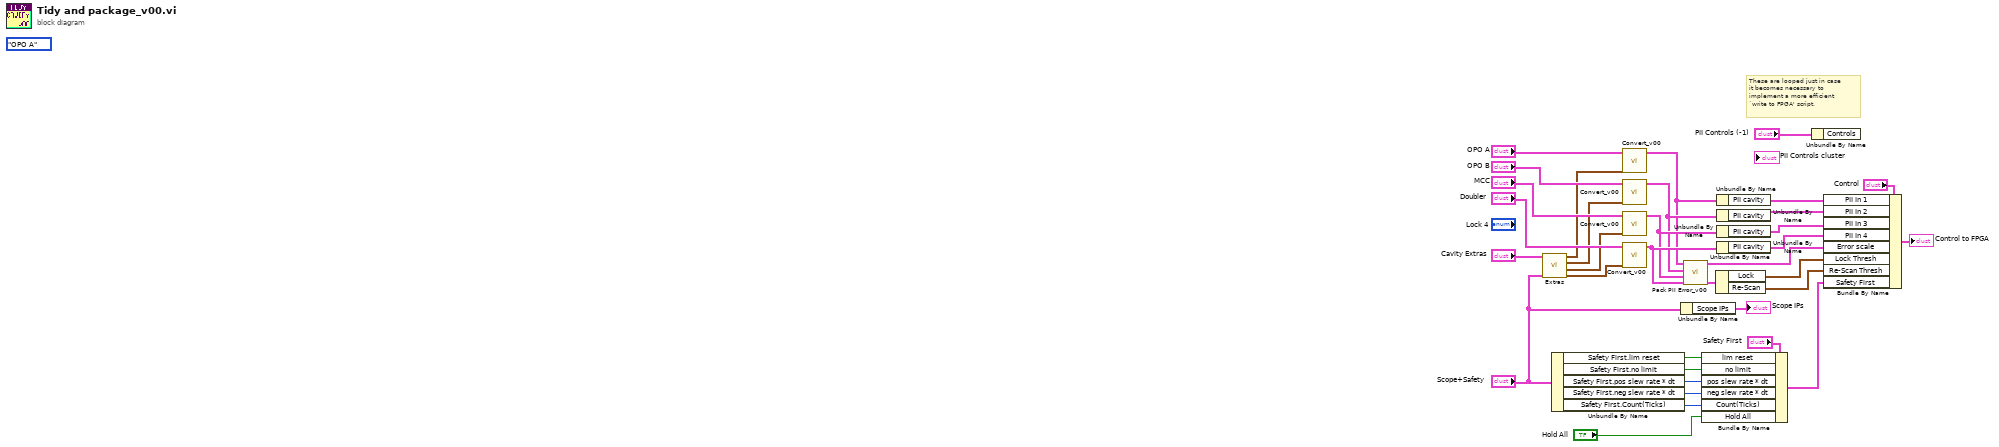
[diagram p0: block diagram]
diagram:
  (unwired) T27."OPO A" ("Tab Control")
  # "These are looped just in case\nit becomes necessary to \nimplement a more efficient \n`write to FPGA' script."
  n1 = call "Extras.vi"("Scope+Safety"="Scope+Safety", "Cavity Extras"="Cavity Extras") -> ("Extras Doubler"=w5:T28, "Extras MCC"=w6:T28, "Extras B"=w7:T28, "Extras A"=w8:T28)  [unwired: 6 in]
  n2 = Unbundle By Name("Scope+Safety") -> ("Safety First.lim reset"=w15:bool, "Safety First.no limit"=w14:bool, "Safety First.pos slew rate * dt"=w13:i16, "Safety First.neg slew rate * dt"=w12:i16, "Safety First.Count(Ticks)"=w11:u32)
  n3 = call "Convert_v00.vi"("Extras PII"=w8, "PII Control"="OPO A") -> ("PII+Error"=w1:T29)  [unwired: 9 in]
  n4 = call "Convert_v00.vi"("Extras PII"=w7, "PII Control"="OPO B") -> ("PII+Error"=w21:T29)  [unwired: 9 in]
  n5 = call "Convert_v00.vi"("Extras PII"=w6, "PII Control"="MCC") -> ("PII+Error"=w22:T29)  [unwired: 9 in]
  n6 = call "Convert_v00.vi"("Extras PII"=w5, "PII Control"="Doubler") -> ("PII+Error"=w23:T29)  [unwired: 9 in]
  n7 = Unbundle By Name("Scope+Safety") -> ("Scope IPs"=→"Scope IPs":T32)
  n8 = call "Pack PII Error_v00.vi"("PII+Error Doubler"=w23, "PII+Error MCC"=w22, "PII+Error B"=w21, "PII+Error A"=w1) -> ("Thresholds"=w29:T33, "Error packed"=w28:T34)  [unwired: 6 in]
  n9 = Bundle By Name(cluster="Safety First", "lim reset"=w15, "no limit"=w14, "pos slew rate * dt"=w13, "neg slew rate * dt"=w12, "Count(Ticks)"=w11, "Hold All"="Hold All") -> (w10:T14)
  n10 = Unbundle By Name(w29) -> ("Lock"=w31:T35, "Re-Scan"=w30:T35)
  n11 = Unbundle By Name(w1) -> ("PII cavity"=w27:T31)
  n12 = Unbundle By Name(w21) -> ("PII cavity"=w24:T31)
  n13 = Unbundle By Name(w22) -> ("PII cavity"=w25:T31)
  n14 = Unbundle By Name(w23) -> ("PII cavity"=w26:T31)
  n15 = Unbundle By Name("PII Controls (-1)") -> ()  [unwired: 1 out]
  n16 = Bundle By Name(cluster="Control", "PII In 1"=w27, "PII In 2"=w24, "PII In 3"=w25, "PII In 4"=w26, "Error scale"=w28, "Lock Thresh"=w31, "Re-Scan Thresh"=w30, "Safety First"=w10) -> (→"Control to FPGA":T18)
